vi "HB_OpenHuskieBoard.vi"(8 "error in (no error)":errorcluster) -> (0 "error out":errorcluster, 3 "HBDeviceRef":T1)   [LabVIEW 2018]
doc: "Opens a serial connection between the roboRIO and the Huskie Board. The user is responsible for synchronizing all access to the Huskie Board."
uses:
  <vilib>/Rock Robotics/WPI/SerialPort/WPI_SerialPortRef.ctl
  <vilib>/Rock Robotics/WPI/SerialPort/WPI_SerialPort.ctl
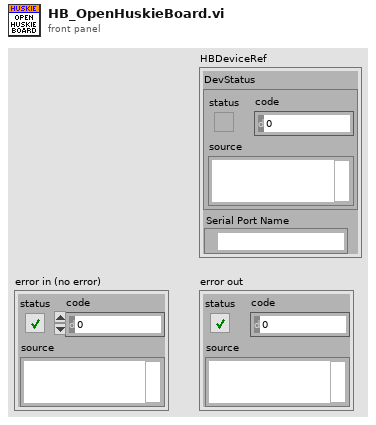
[diagram p1: front panel]
types:
  T1 = typedef "WPI_SerialPortRef.ctl" = cluster{"DevStatus":errorcluster, "Serial Port Name":refnum<visa-resource-name>}
  T2 = typedef "WPI_SerialPort.ctl" = enum16{"Onboard RS-232", "MXP TTL", "USB 1", "USB 2"}
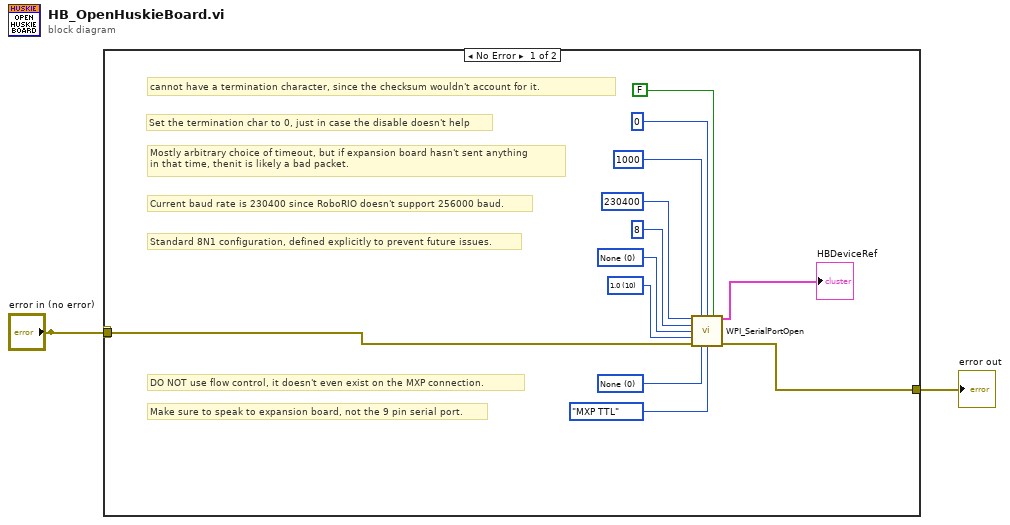
[diagram p0: block diagram]
diagram:
  n1 = case shown="No Error" "error in (no error)" {
    selector: "error in (no error)" -> [_ w15]
    tunnel: [w13 w15] -> w2
    tunnel: "error in (no error)" -> [w9 _]
    frame No Error {
      w11 = u16 10 items=["1.0"=10, "1.5"=15, "2.0"=20] ("Stop Bits")
      w6 = u16 0 items=["None", "XON/XOFF", "RTS/CTS", "XON/XOFF & RTS/CTS", "DTR/DSR", "XON/XOFF & DTR/DSR"] ("Flow Control")
      w5 = u16 0 items=["None", "Odd", "Even", "Mark", "Space"] ("Parity")
      # "Make sure to speak to expansion board, not the 9 pin serial port."
      # "DO NOT use flow control, it doesn't even exist on the MXP connection."
      # "Standard 8N1 configuration, defined explicitly to prevent future issues."
      # "Current baud rate is 230400 since RoboRIO doesn't support 256000 baud."
      # "Mostly arbitrary choice of timeout, but if expansion board hasn't sent anything\nin that time, thenit is likely a bad packet."
      # "Set the termination char to 0, just in case the disable doesn't help"
      # "cannot have a termination character, since the checksum wouldn't account for it."
      n2 = call <vilib>:"WPI_SerialPortOpen.vi"("Baud Rate"=u32 230400, "Timeout Value (ms)"=u32 1000, "Termination Char (0xA = '\\n' = LF)"=u8 0 ("Termination Char (0xA = '\\n' = LF)"), "Enable Termination Char? (T)"=FALSE, "Data Bits"=u16 8, "Parity"=w5, "Stop Bits"=w11, "error in (no error)"=w9, "Flow Control"=w6, "Serial Port"=WPI_SerialPort."MXP TTL") -> ("SerialPortRef"=→"HBDeviceRef":T1, "error out"=w13:errorcluster)  [unwired: 4 in]
    }
    frame Error {
    }
  }
  "error out" <- w2
